vi "CSM - Module VI Reference.vi"(6 "Response Timeout(5000ms)":i32=5000, 7 "Current Module(\"\" to generate a ID)":string, 8 "error in (no error)":errorcluster, 11 "CSM":string) -> (0 "error out":errorcluster, 3 "CSM Module VIRef":refnum<vi>)   [LabVIEW 2020, in "Communicable State Machine.lvlib"]
uses:
  Communicable State Machine.lvlib
  Priority Queue.lvclass/Priority Queue.ctl
  CSMP-Sync Call.vi
  uuid.vi
  Build Error Cluster.vi
  Trim Both Whitespace.vi
  _CSMObj-Message Check.vi
  _CSMObj-Enqueue Cross-Module Message.vi
  _CSMOFGV Get.vi
  Enqueue Element.vi
  CSM No Target Error.vi
  _CSMOFGV.vi
  CSM Not Allowed Message.vi
  CSM Target Error.vi
  CSM Unhandled State Error.vi
  CSM Target Timeout Error.vi
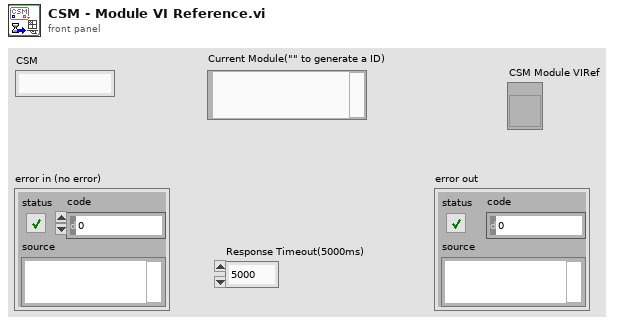
[diagram p1: front panel]
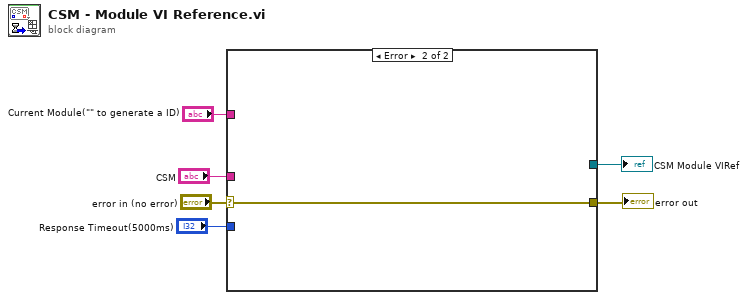
[diagram p0: block diagram]
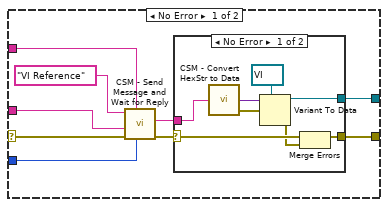
[diagram p2: hidden frame]
diagram:
  n1 = case shown="Error" "error in (no error)" {
    selector: "error in (no error)" -> [w15 w25]
    tunnel: "Response Timeout(5000ms)" -> [w14 _]
    tunnel: "CSM" -> [w10 _]
    tunnel: [w9 w25] -> w3
    tunnel: "Current Module(\"\" to generate a ID)" -> [w8 _]
    tunnel: [w7 _] -> w1
    frame No Error {
      n2 = call "CSM - Send Message and Wait for Reply.vi"("Response Timeout(5000ms)"=w14, "Current Module(\"\" to generate a ID)"=w8, "Error In (no error)"=w15, "Target Module"=w10, "State"="VI Reference") -> ("error out"=w12:errorcluster, "Response"=w11:string)  [unwired: 4 in, 1 out]
      n3 = case shown="No Error" w12 {
        selector: w12 -> [w18 w24]
        tunnel: w11 -> [w23 _]
        tunnel: [w19 w24] -> w9
        tunnel: [w16 _] -> w7
        frame No Error {
          n4 = call "CSM - Convert HexStr to Data.vi"("HEX String"=w23) -> ("Variant"=w21:variant, "error out"=w22:errorcluster)  [unwired: 7 in]
          n5 = Variant To Data(error in=w22, type=refnum<vi> refnum ("Current VI Reference"), Variant=w21) -> (data=w16:refnum<vi>, error out=w17:errorcluster)
          n6 = Merge Errors(w18, w17) -> (w19:errorcluster)
        }
        frame Error {
        }
      }
    }
    frame Error {
    }
  }
  "error out" <- w3
  "CSM Module VIRef" <- w1
